vi "CRYFlatten Signal Generator.vi"(11 "Signal Gen'r settings":T1={"gen'r mode"=0, "frequency"=0, "output level"=0.0, "wave path"="", "wav play mode"=0, "duration"=0.0, "n times"=0, "channel"=0, "wav level"=0.0, "EQ"=FALSE, "f knob log"=FALSE, "f knob low"=0.0, "f knob high"=0.0, "ol knob log"=FALSE, "ol knob low"=0.0, "ol knob high"=0.0, "Lin Display Prefs"="%#_6p", "dB Display Prefs"="%.1f", "Duration noise"=20.0, "Min freq noise"=20.0, "Max freq noise"=20000.0, "Channel String"="", "Play Sine Wave"=0} {"Duration noise" format="%.2f"; "Max freq noise" format="%.2f"; "Min freq noise" format="%.2f"; "ol knob high" format="%.2f"; "ol knob low" format="%.2f"; "f knob high" format="%.2f"; "f knob low" format="%.2f"; "wav level" format="%.2f"; "duration" format="%.2f"; "output level" format="%.2f"}) -> (3 "Flat Signal Gen'r settings":string="%#_6p")   [LabVIEW 2013]
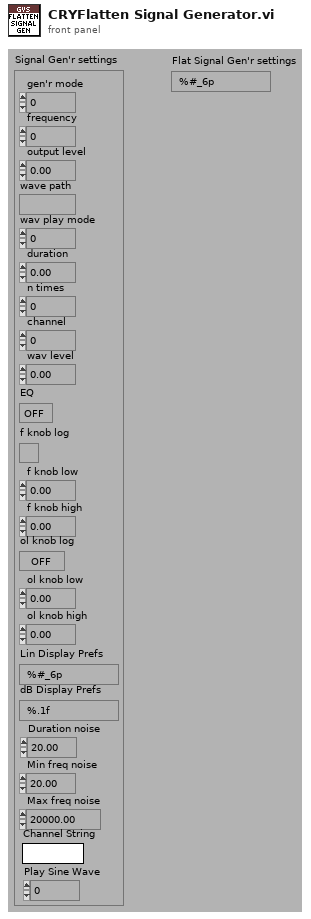
[diagram p1: front panel]
types:
  T1 = cluster{"gen'r mode":i32, "frequency":u32, "output level":dbl, "wave path":string, "wav play mode":i32, "duration":dbl, "n times":i32, "channel":i32, "wav level":dbl, "EQ":bool, "f knob log":bool, "f knob low":dbl, "f knob high":dbl, "ol knob log":bool, "ol knob low":dbl, "ol knob high":dbl, "Lin Display Prefs":string, "dB Display Prefs":string, "Duration noise":dbl, "Min freq noise":dbl, "Max freq noise":dbl, "Channel String":string, "Play Sine Wave":i32}
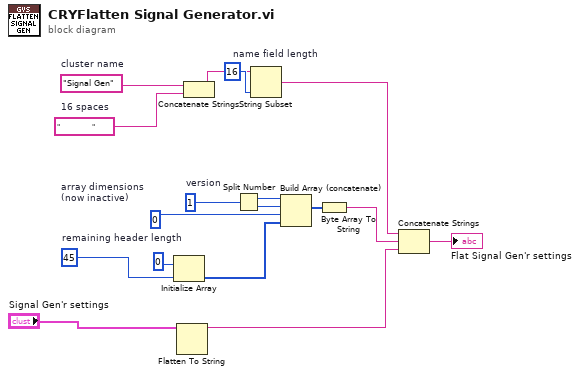
[diagram p0: block diagram]
diagram:
  w4 = u8 0  # array dimensions (now inactive)
  w7 = 16  # name field length
  w8 = "                "  # 16 spaces
  w9 = "Signal Gen"  # cluster name
  w13 = 45  # remaining header length
  w17 = u16 1  # version
  n1 = Initialize Array(u8 0, w13) -> (w10:u8[])
  n2 = Flatten To String(anything="Signal Gen'r settings") -> (data string=w3:string)  [unwired: 1 in, 4 out]
  n3 = Concatenate Strings(w9, w8) -> (w6:string)
  n4 = Split Number(x=w17) -> (hi(x)=w16:u8, lo(x)=w15:u8)
  n5 = String Subset(string=w6, length (rest)=w7) -> (substring=w5:string)  [unwired: 1 out]
  n6 = Build Array (concatenate)(w16, w15, w4, w10) -> (w12:u8[])
  n7 = Byte Array To String(unsigned byte array=w12) -> (string=w11:string)
  n8 = Concatenate Strings(w5, w11, w3) -> (→"Flat Signal Gen'r settings":string)
